vi "Telnet_Close.vi"(8 "error in (no error)":errorcluster, 11 "connection ID In":refnum<k5>) -> (0 "error out":errorcluster)   [LabVIEW 2018]
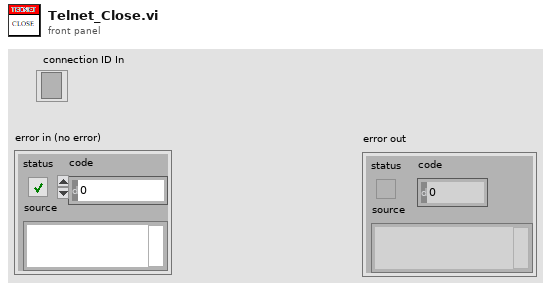
[diagram p1: front panel]
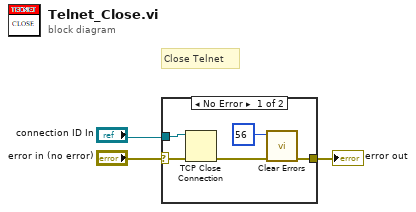
[diagram p0: block diagram]
diagram:
  # "Close Telnet"
  n1 = case shown="No Error" "error in (no error)" {
    selector: "error in (no error)" -> [w4 w9]
    tunnel: "connection ID In" -> [w8 _]
    tunnel: [w5 w9] -> w2
    frame No Error {
      n2 = TCP Close Connection(connection ID=w8, error in (no error)=w4) -> (error out=w6:errorcluster)  [unwired: 1 in, 1 out]
      n3 = call "Clear Errors.vi"("error in (no error)"=w6, "specific error code to clear (0: all)"=56) -> ("error out"=w5:errorcluster)  [unwired: 4 in, 1 out]
    }
    frame Error {
    }
  }
  "error out" <- w2
